vi "D-O Settings Dialog.vi"(8 "error in (no error)":errorcluster, 10 "Message Queues":T6, 11 "D-O Module State Cluster In":T2={"D-O Module Config"={"GUID"="", "Drop Coords"={"Horizontal"=0, "Vertical"=0}, "Process Name"="", "Settings"={"DAQmx Task Name"="", "Output Channel"=0, "Time On (Sec)"=0.0, "Time Off (Sec)"=0.0, "Output Channel Names"=[], "Run?"=FALSE}, "Load Count"=0}, "State"=enum."Idle", "Start Time"=timestamp(0 s since 1904-01-01), "Current Time"=timestamp(0 s since 1904-01-01), "First Iteration"=FALSE, "Data"={"Valve State"={"DAQmx Task Name"="", "Output Channel"=0, "Time On (Sec)"=0.0, "Time Off (Sec)"=0.0, "Output Channel Names"=[], "Run?"=FALSE}}, "Process Name"="", "Program On?"=FALSE} {"Data"."Valve State"."Output Channel" items=["Choose a Channel"]; "D-O Module Config"."Settings"."Output Channel" items=["Choose a Channel"]}) -> (0 "error out":errorcluster, 1 "Cancelled?":bool=TRUE, 2 "UI Refresh Needed?":bool, 3 "D-O Module Config Out":T3 {"Settings"."Output Channel" items=["Choose a Channel"]})   [LabVIEW 2018, in "D-O Module.lvlib"]
doc: "Dialog for selecting user specified settings."
uses:
  D-O Module.lvlib
  All Message Queues.ctl
  support/Message Queue/Message Cluster.ctl
  D-O Module Config Cluster.ctl
  <vilib>/Utility/miscctls.llb/LVPoint32TypeDef.ctl
  D-O Module Settings Cluster.ctl
  D-O Module State Cluster.ctl
  Measure Instrument/State Enum.ctl
  support/Message Queue/Enqueue Message (Single).vi
  <vilib>/Utility/xml.llb/Write to XML File(string).vi
  Settings/Settings.lvlib
  <resource>/objmgr/daqmx.rc
  support/Message Queue/Message Queue.lvlib
  Measure Instrument/Feed Module Engine.lvlib
panel:
  in  "Module Name":string
  out "Channels":string[](array[string])
  in  "D-O Settings":T1 {"Output Channel" items=["Choose a Channel", "Card 1 Channel 0", "Card 1 Channel 1", "Card 1 Channel 2", "Card 1 Channel 3", "Card 1 Channel 4", "Card 1 Channel 5", "Card 1 Channel 6", "Card 1 Channel 7", "Card 2 Channel 0", "Card 2 Channel 1", "Card 2 Channel 2", "Card 2 Channel 3", "Card 2 Channel 4", "Card 2 Channel 5", "Card 2 Channel 6", "Card 2 Channel 7"]}
  in  "Start":bool
  in  "Stop":bool
  in  "Cancel Button":bool
  in  "OK Button":bool
  # "Non visible portion of dialog (needed for connector pane)."
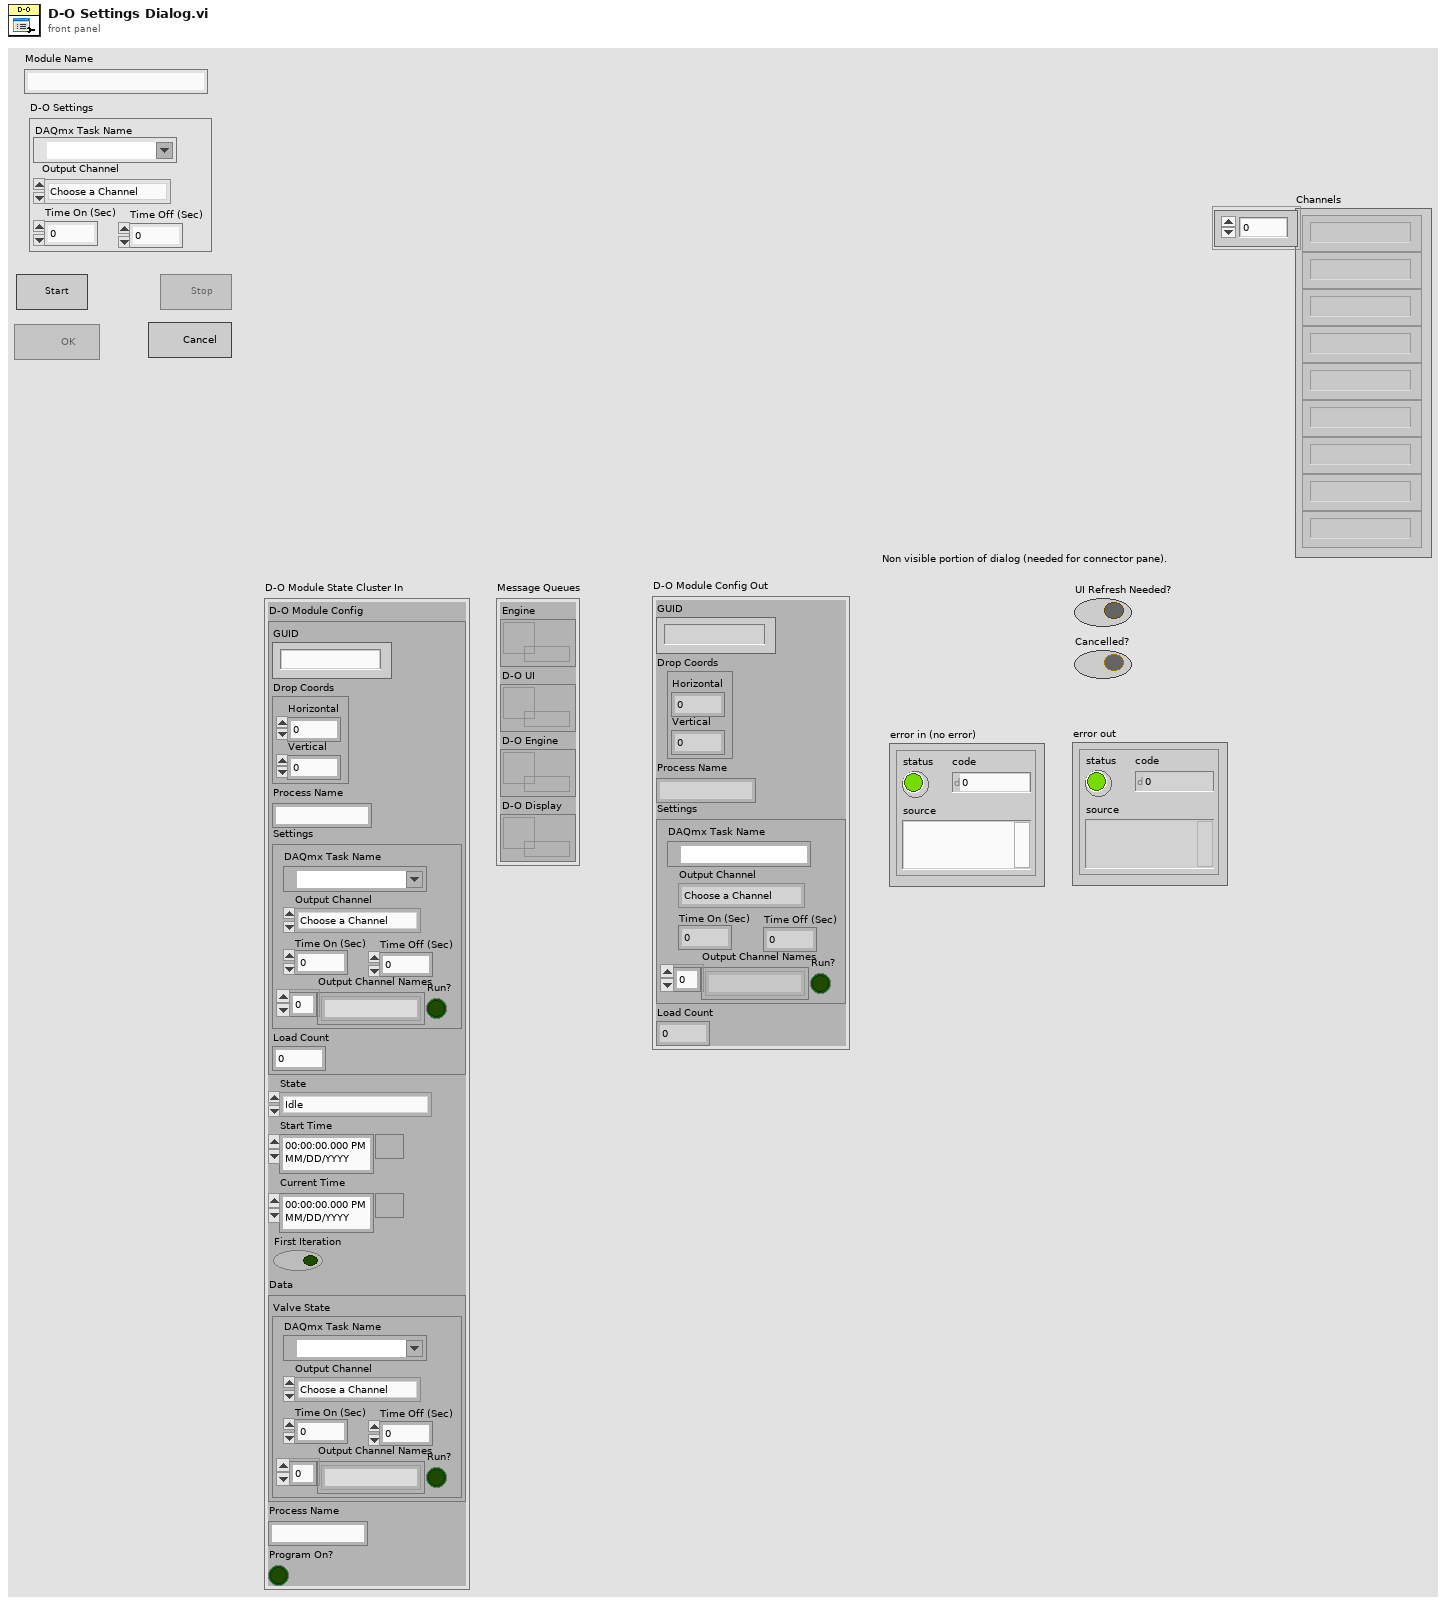
[diagram p1: front panel]
types:
  T1 = typedef "D-O Module.lvlib/D-O Module Settings Cluster.ctl" = cluster{"DAQmx Task Name":refnum<k21>, "Output Channel":u16, "Time On (Sec)":dbl, "Time Off (Sec)":dbl, "Output Channel Names":string[], "Run?":bool}
  T2 = typedef "D-O Module.lvlib/D-O Module State Cluster.ctl" = cluster{"D-O Module Config":T3, "State":T5, "Start Time":timestamp, "Current Time":timestamp, "First Iteration":bool, "Data":cluster{"Valve State":T1}, "Process Name":string, "Program On?":bool}
  T3 = typedef "D-O Module.lvlib/D-O Module Config Cluster.ctl" = cluster{"GUID":string, "Drop Coords":T4, "Process Name":string, "Settings":T1, "Load Count":i32}
  T4 = typedef "LVPoint32TypeDef.ctl" = cluster{"Horizontal":i32, "Vertical":i32}
  T5 = typedef "Feed Module.lvlib/Feed Module Engine.lvlib/State Enum.ctl" = enum16{"Measuring", "Idle", "Paused"}
  T6 = typedef "D-O Module.lvlib/All Message Queues.ctl" = cluster{"Engine":refnum<queue>, "D-O UI":refnum<queue>, "D-O Engine":refnum<queue>, "D-O Display":refnum<queue>}
  T7 = enum8{"Enabled", "Disabled", "Disabled and Grayed Out"}
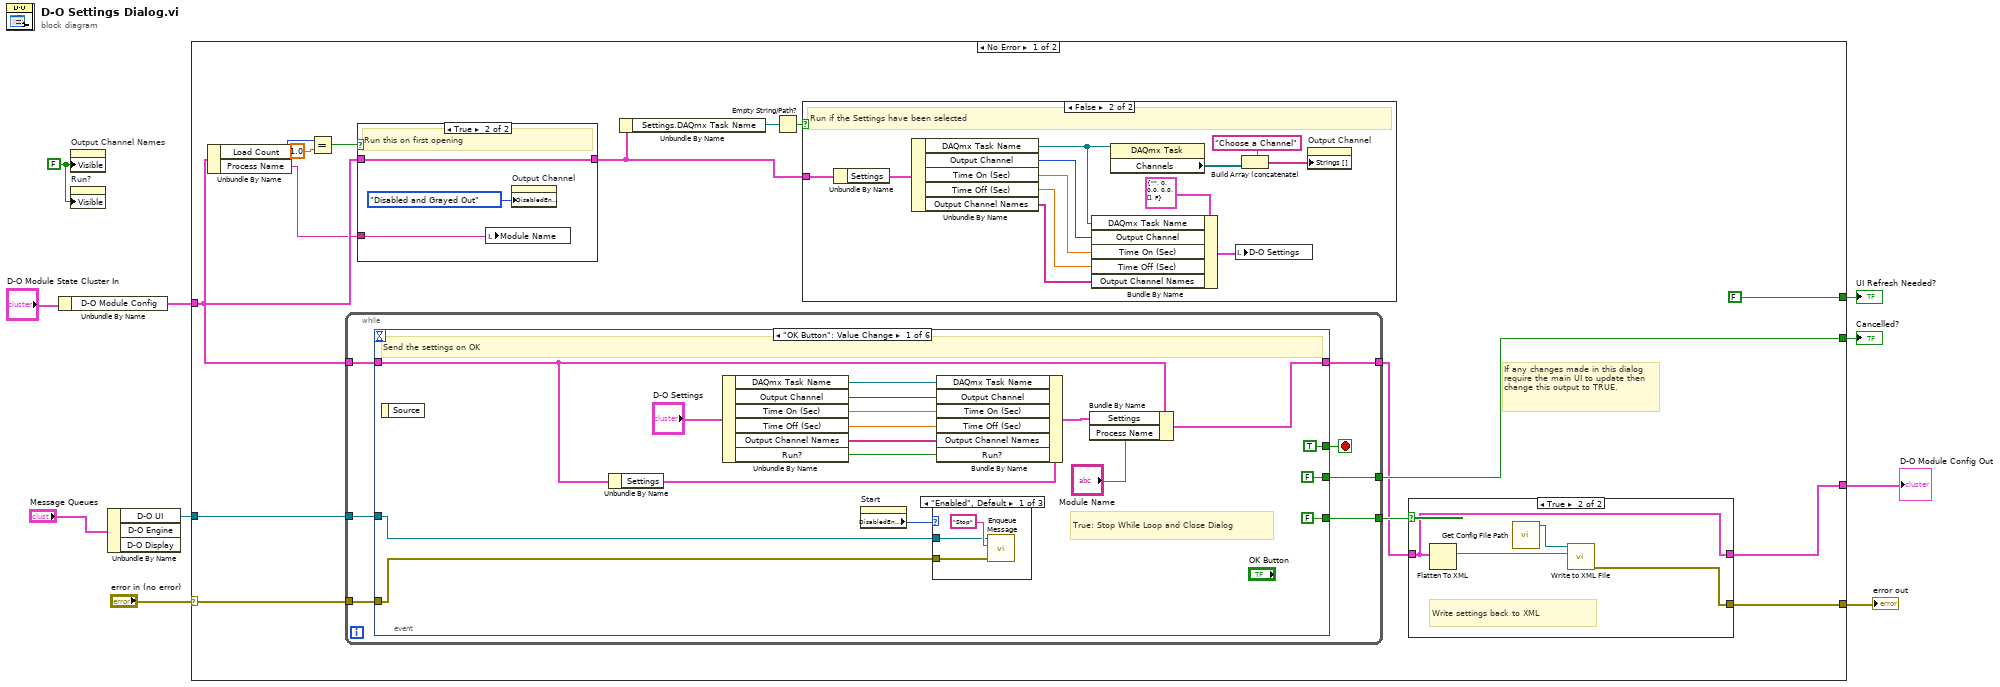
[diagram p0: block diagram]
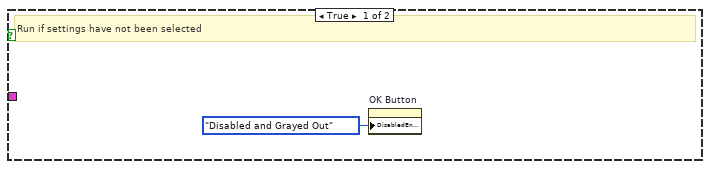
[diagram p2: hidden frame]
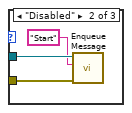
[diagram p4: hidden frame]
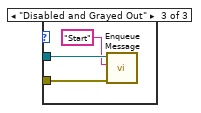
[diagram p5: hidden frame]
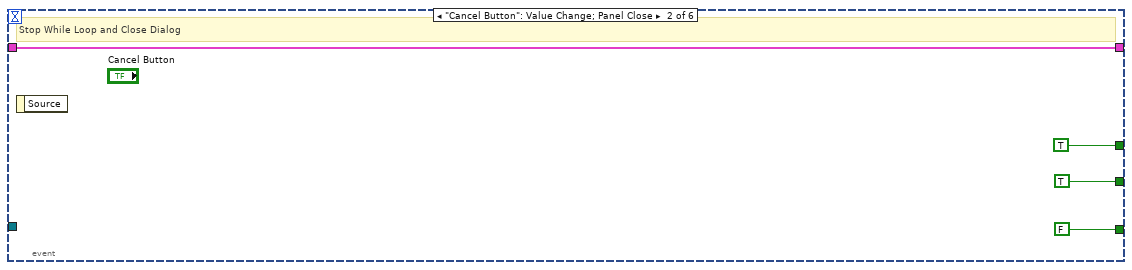
[diagram p6: hidden frame]
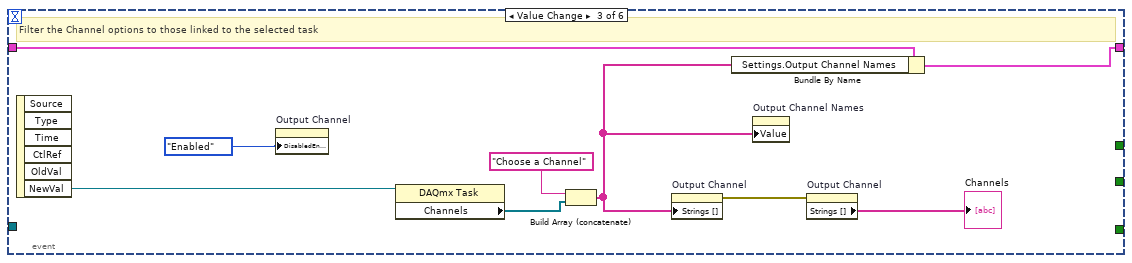
[diagram p7: hidden frame]
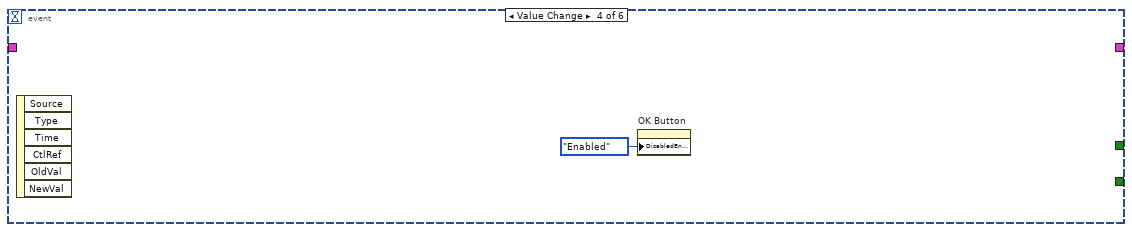
[diagram p8: hidden frame]
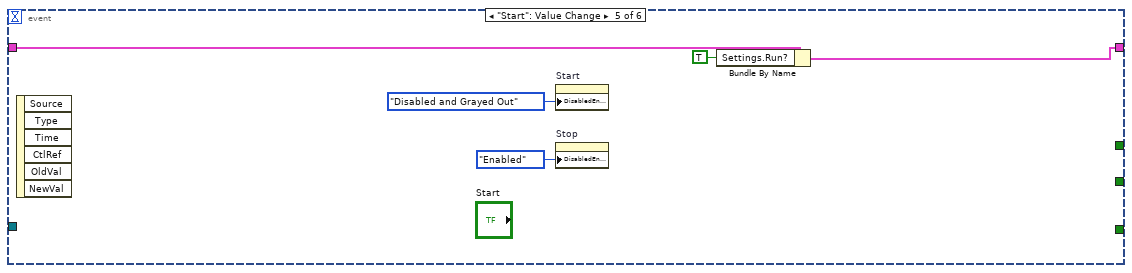
[diagram p9: hidden frame]
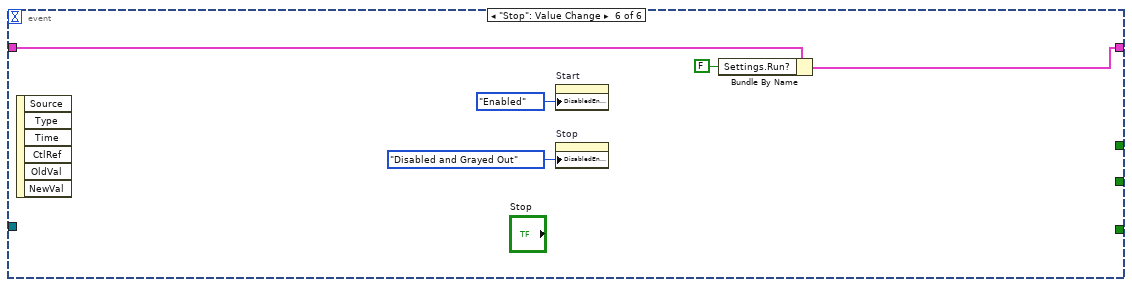
[diagram p10: hidden frame]
diagram:
  w1 = FALSE ("Visible")
  n1 = Unbundle By Name("D-O Module State Cluster In") -> ("D-O Module Config"=w2:T3)
  n2 = property on="Output Channel Names" class="Arr (strict)"("Visible"=w1) -> ()  [unwired: 2 in, 2 out]
  n3 = property on="Run?" class="Bool (strict)"("Visible"=w1) -> ()  [unwired: 2 in, 2 out]
  n4 = Unbundle By Name("Message Queues") -> ("D-O UI"=w7:refnum<queue>)  [unwired: 2 out]
  n5 = case shown="No Error" "error in (no error)" {
    selector: "error in (no error)" -> [w21 w109]
    tunnel: [w23 w109] -> w10
    tunnel: w2 -> [w12 w107]
    tunnel: [w24 w107] -> w4
    tunnel: [FALSE ("UI Refresh Needed?") _] -> w9
    tunnel: [w25 TRUE ("UI Refresh Needed?")] -> w8
    tunnel: w7 -> [w22 _]
    frame No Error {
      # "If any changes made in this dialog require the main UI to update then change this output to TRUE."
      n6 = Unbundle By Name(w12) -> ("Load Count"=w20:i32, "Process Name"=w11:string)
      n7 = Equal?(x=w20, y=1.0) -> (x = y?=w17:bool)
      n8 = while {
        tunnel: [w50] -> w16
        tunnel: [w48] -> w25
        tunnel: w22 -> [w46]
        tunnel: w21 -> [w45]
        tunnel: w12 -> [w44]
        tunnel: [w47] -> w15
        stop <- w49 stop-if-true
        n9 = event shown="[0] \"OK Button\": Value Change" {
          selector: _ -> [_ _ _ _ _ _]
          dyn-events: _ -> [_ _ _ _ _ _]
          timeout: _ -> [_ _ _ _ _ _]
          tunnel: [FALSE ("UI Refresh Needed?") FALSE ("UI Refresh Needed?") _ _ _ _] -> w50
          tunnel: [TRUE TRUE _ _ _ _] -> w49
          tunnel: [FALSE ("UI Refresh Needed?") TRUE ("UI Refresh Needed?") _ _ _ _] -> w48
          tunnel: w44 -> [w64 w78 w84 _ w94 w98]
          tunnel: [w62 w78 w83 _ w93 w97] -> w47
          tunnel: w46 -> [w57 _ _ _ _ _]
          tunnel: w45 -> [w56 _ _ _ _ _]
          event "OK Button": Value Change {
            # "True: Stop While Loop and Close Dialog"
            # "Send the settings on OK"
            n10 = event-data() -> ()  [unwired: 1 in, 1 out]
            n11 = Unbundle By Name(w64) -> ("Settings"=w65:T1)
            n12 = Unbundle By Name("D-O Settings") -> ("DAQmx Task Name"=w61:refnum<k21>, "Output Channel"=w60:u16, "Time On (Sec)"=w59:dbl, "Time Off (Sec)"=w58:dbl, "Output Channel Names"=w53:string[], "Run?"=w52:bool)
            n13 = property on="Start" class="Bool"() -> ("DisabledEnum"=w55:T7)  [unwired: 2 in, 2 out]
            n14 = case shown="\"Enabled\", Default" w55 {
              tunnel: w57 -> [w70 w74 w77]
              tunnel: w56 -> [w69 w73 w76]
              frame "Enabled", Default {
                n15 = call-poly "Enqueue Message.vi"("error in (no error)"=w69, "Message"="Stop", "Message Queue"=w70) -> ()  [unwired: 7 in, 2 out]
              }
              frame "Disabled" {
                n16 = call-poly "Enqueue Message.vi"("error in (no error)"=w73, "Message"="Start", "Message Queue"=w74) -> ()  [unwired: 7 in, 2 out]
              }
              frame "Disabled and Grayed Out" {
                n17 = call-poly "Enqueue Message.vi"("error in (no error)"=w76, "Message"="Start", "Message Queue"=w77) -> ()  [unwired: 7 in, 2 out]
              }
            }
            n18 = Bundle By Name(cluster=w65, "DAQmx Task Name"=w61, "Output Channel"=w60, "Time On (Sec)"=w59, "Time Off (Sec)"=w58, "Output Channel Names"=w53, "Run?"=w52) -> (w63:T1)
            n19 = Bundle By Name(cluster=w64, "Settings"=w63, "Process Name"="Module Name") -> (w62:T3)
          }
          event "Cancel Button": Value Change; Panel Close {
            # "Stop While Loop and Close Dialog"
            n20 = event-data() -> ()  [unwired: 1 in, 1 out]
          }
          event Value Change {
            # "Filter the Channel options to those linked to the selected task"
            n21 = event-data() -> ("NewVal"=w90:refnum<k21>)  [unwired: 1 in, 5 out]
            n22 = property on="Output Channel" class="Ring (strict)"("DisabledEnum"=T7."Enabled" ("Disabled")) -> ()  [unwired: 2 in, 2 out]
            n23 = property class="DAQmx Task"(reference=w90) -> ("Channels"=w88:refnum<k21>[])  [unwired: 1 in, 2 out]
            n24 = Build Array (concatenate)("Choose a Channel", w88) -> (w82:string[])
            n25 = property on="Output Channel" class="Ring (strict)"("Strings []"=w82) -> (error out=w86:errorcluster)  [unwired: 2 in, 1 out]
            n26 = Bundle By Name(cluster=w84, "Settings.Output Channel Names"=w82) -> (w83:T3)
            n27 = property on="Output Channel Names" class="Arr (strict)"("Value"=w82) -> ()  [unwired: 2 in, 2 out]
            n28 = property on="Output Channel" class="Ring (strict)"(error in=w86) -> ("Strings []"=→"Channels":string[])  [unwired: 1 in, 2 out]
          }
          event Value Change {
            n29 = event-data() -> ()  [unwired: 1 in, 6 out]
            n30 = property on="OK Button" class="Bool"("DisabledEnum"=T7."Enabled" ("Disabled")) -> ()  [unwired: 2 in, 2 out]
          }
          event "Start": Value Change {
            n31 = event-data() -> ()  [unwired: 1 in, 6 out]
            n32 = property on="Start" class="Bool"("DisabledEnum"=T7."Disabled and Grayed Out" ("Disabled")) -> ()  [unwired: 2 in, 2 out]
            n33 = property on="Stop" class="Bool"("DisabledEnum"=T7."Enabled" ("Disabled")) -> ()  [unwired: 2 in, 2 out]
            n34 = Bundle By Name(cluster=w94, "Settings.Run?"=TRUE) -> (w93:T3)
          }
          event "Stop": Value Change {
            n35 = event-data() -> ()  [unwired: 1 in, 6 out]
            n36 = property on="Start" class="Bool"("DisabledEnum"=T7."Enabled" ("Disabled")) -> ()  [unwired: 2 in, 2 out]
            n37 = property on="Stop" class="Bool"("DisabledEnum"=T7."Disabled and Grayed Out" ("Disabled")) -> ()  [unwired: 2 in, 2 out]
            n38 = Bundle By Name(cluster=w98, "Settings.Run?"=FALSE) -> (w97:T3)
          }
        }
      }
      n39 = case shown="True" w17 {
        tunnel: w12 -> [w40 w43]
        tunnel: [w40 w43] -> w18
        tunnel: w11 -> [_ w41]
        frame False {
        }
        frame True {
          # "Run this on first opening"
          n40 = local write "Module Name"(w41) -> ()
          n41 = property on="Output Channel" class="Ring (strict)"("DisabledEnum"=T7."Disabled and Grayed Out" ("Disabled")) -> ()  [unwired: 2 in, 2 out]
        }
      }
      n42 = Unbundle By Name(w18) -> ("Settings.DAQmx Task Name"=w14:refnum<k21>)
      n43 = Empty String/Path?(string/path=w14) -> (empty?=w13:bool)
      n44 = case shown="False" w13 {
        tunnel: w18 -> [_ w38]
        frame True {
          # "Run if settings have not been selected"
          n45 = property on="OK Button" class="Bool"("DisabledEnum"=T7."Disabled and Grayed Out" ("Disabled")) -> ()  [unwired: 2 in, 2 out]
        }
        frame False {
          # "Run if the Settings have been selected"
          n46 = Unbundle By Name(w38) -> ("Settings"=w39:T1)
          n47 = Unbundle By Name(w39) -> ("DAQmx Task Name"=w33:refnum<k21>, "Output Channel"=w37:u16, "Time On (Sec)"=w36:dbl, "Time Off (Sec)"=w35:dbl, "Output Channel Names"=w28:string[])
          n48 = Bundle By Name(cluster=T1 {"DAQmx Task Name"="", "Output Channel"=0, "Time On (Sec)"=0.0, "Time Off (Sec)"=0.0, "Output Channel Names"=[], "Run?"=FALSE} ("D-O Settings"), "DAQmx Task Name"=w33, "Output Channel"=w37, "Time On (Sec)"=w36, "Time Off (Sec)"=w35, "Output Channel Names"=w28) -> (w34:T1)
          n49 = property class="DAQmx Task"(reference=w33) -> ("Channels"=w31:refnum<k21>[])  [unwired: 1 in, 2 out]
          n50 = local write "D-O Settings"(w34) -> ()
          n51 = Build Array (concatenate)("Choose a Channel", w31) -> (w30:string[])
          n52 = property on="Output Channel" class="Ring (strict)"("Strings []"=w30) -> ()  [unwired: 2 in, 2 out]
        }
      }
      n53 = case shown="True" w16 {
        tunnel: w15 -> [w102 w103]
        tunnel: [_ w104] -> w23
        tunnel: [w102 w103] -> w24
        frame False {
        }
        frame True {
          # "Write settings back to XML"
          n54 = Flatten To XML(anything=w103) -> (xml string=w105:string)
          n55 = call "Get Config File Path.vi"() -> ("XML File Path"=w106:path)  [unwired: 10 in, 1 out]
          n56 = call-poly <vilib>:"Write to XML File.vi"("XML Input"=w105, "XML File Path"=w106) -> ("error out"=w104:errorcluster)  [unwired: 7 in, 2 out]
        }
      }
    }
    frame Error {
    }
  }
  "UI Refresh Needed?" <- w9
  "error out" <- w10
  "Cancelled?" <- w8
  "D-O Module Config Out" <- w4
